vi "Main.vi"() -> ()   [LabVIEW 2015]
uses:
  TypDefs/Loop States.ctl
  TypDefs/Loop Data.ctl
panel:
  in  "device name":tag="myDAQ1"
  in  "Exit Button":bool
  in  "Start Button":bool
  out "Status":string
  in  "Clear Button":bool
  in  "Save Button":bool
  out "XY Graph":cluster{"X":dbl[], "Y":dbl[]}(graph)
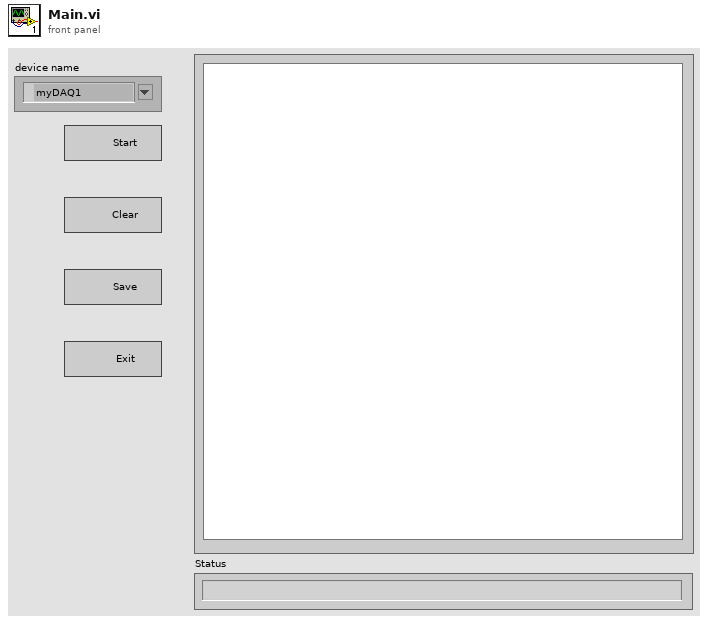
[diagram p1: front panel]
types:
  T1 = typedef "Loop Data.ctl" = cluster{"Status":string, "Graph Data":cluster{"X":dbl[], "Y":dbl[]}, "Recording Status":bool}
  T2 = typedef "Loop States.ctl" = enum16{"Error", "Wait for events", "Measure positions", "Update UI", "Initialization"}
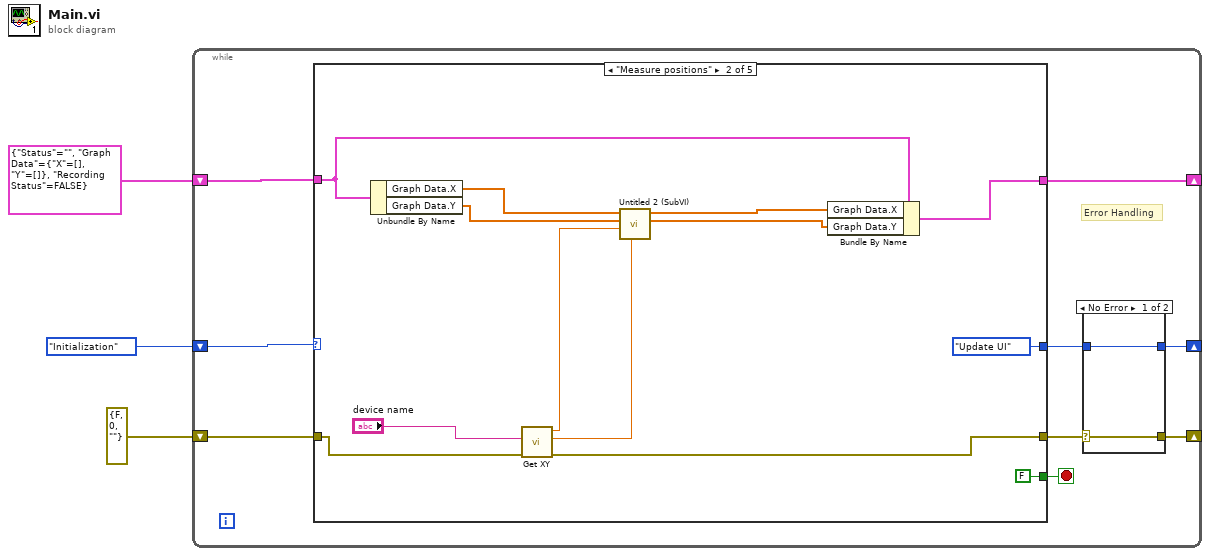
[diagram p0: block diagram]
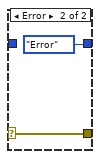
[diagram p2: hidden frame]
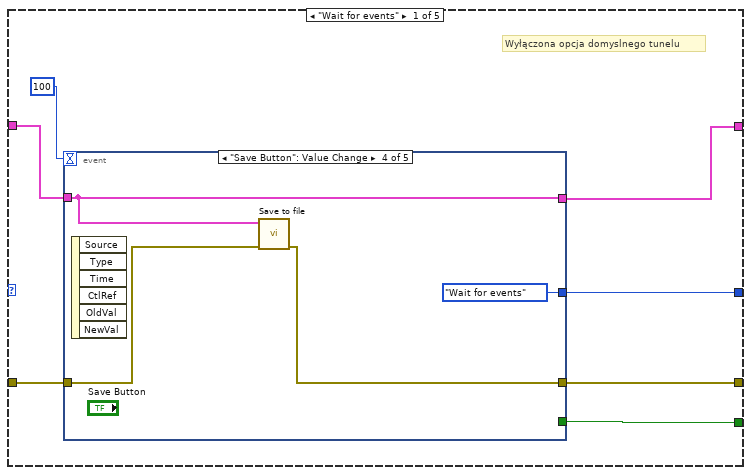
[diagram p3: hidden frame]
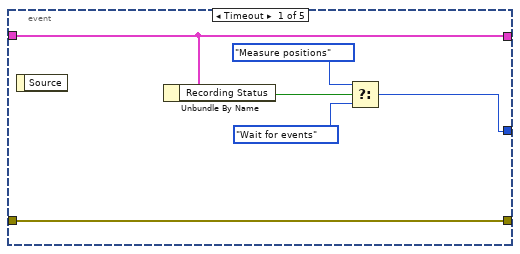
[diagram p4: hidden frame]
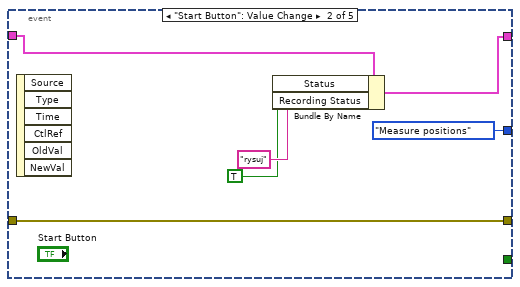
[diagram p5: hidden frame]
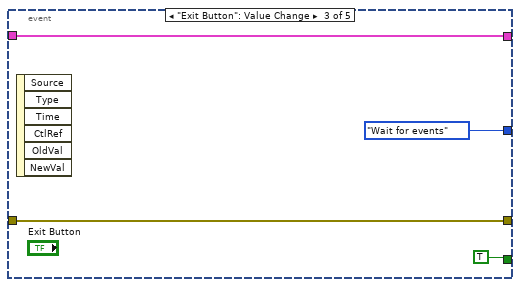
[diagram p6: hidden frame]
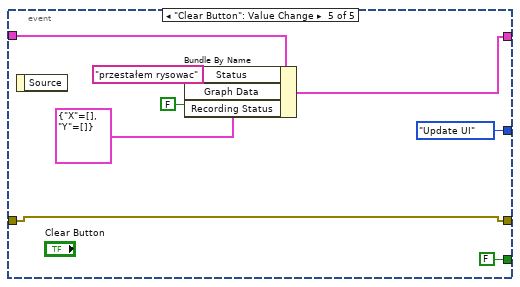
[diagram p7: hidden frame]
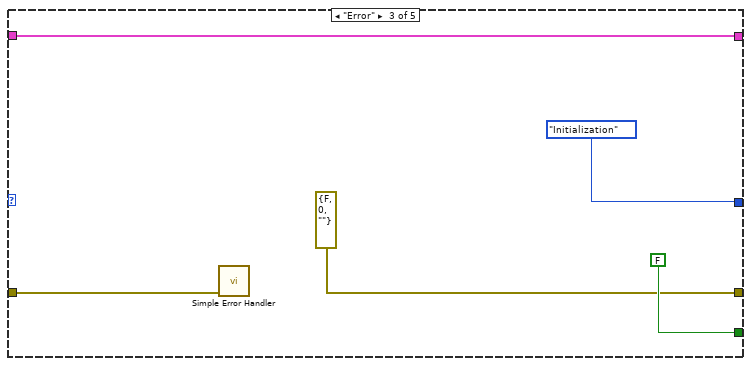
[diagram p8: hidden frame]
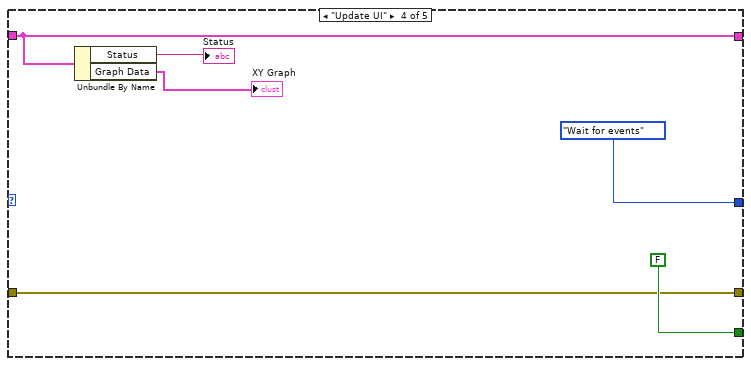
[diagram p9: hidden frame]
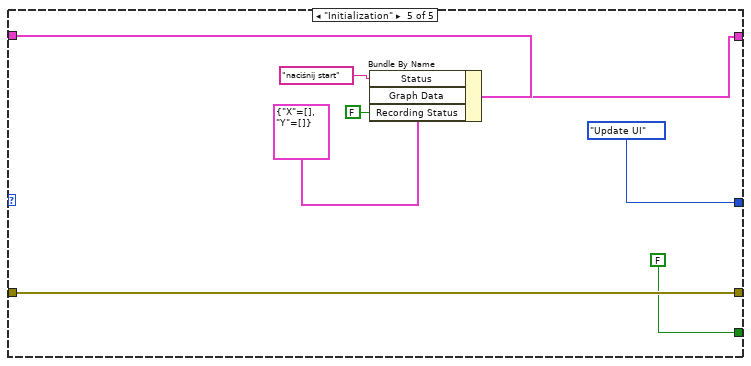
[diagram p10: hidden frame]
diagram:
  n1 = while {
    shift-right: [w10] -> _
    shift-left: T1 {"Status"="", "Graph Data"={"X"=[], "Y"=[]}, "Recording Status"=FALSE} -> [w11]
    shift-right: [w5] -> _
    shift-left: Loop_States."Initialization" -> [w12]
    shift-right: [w4] -> _
    shift-left: errorcluster {"status"=FALSE, "code"=0, "source"=""} ("error constant") -> [w8]
    stop <- w9 stop-if-true
    # "Error Handling"
    n2 = case shown="\"Measure positions\"" w12 {
      tunnel: w11 -> [w22 w61 w66 w71 w83]
      tunnel: [w20 w63 w66 w71 w82] -> w10
      tunnel: [w19 FALSE FALSE FALSE FALSE] -> w9
      tunnel: [w21 Loop_States."Update UI" Loop_States."Initialization" Loop_States."Wait for events" Loop_States."Update UI"] -> w6
      tunnel: w8 -> [w18 w60 w68 w74 w77]
      tunnel: [w17 w59 errorcluster {"status"=FALSE, "code"=0, "source"=""} ("error constant") w74 w77] -> w7
      frame "Wait for events" {
        # "Wyłączona opcja domyslnego tunelu"
        n3 = event shown="[3] \"Save Button\": Value Change" {
          selector: _ -> [_ _ _ _ _]
          dyn-events: _ -> [_ _ _ _ _]
          timeout: 100 -> [_ _ _ _ _]
          tunnel: w22 -> [w24 w35 w38 w42 w51]
          tunnel: [w25 Loop_States."Measure positions" Loop_States."Wait for events" Loop_States."Wait for events" Loop_States."Update UI"] -> w21
          tunnel: [w24 w31 w38 w42 w50] -> w20
          tunnel: [_ _ TRUE _ FALSE] -> w19
          tunnel: w18 -> [w29 w32 w36 w41 w45]
          tunnel: [w29 w32 w36 w40 w45] -> w17
          event Timeout {
            n4 = event-data() -> ()  [unwired: 1 in, 1 out]
            n5 = Unbundle By Name(w24) -> ("Recording Status"=w28:bool)
            n6 = Select(t=Loop_States."Measure positions", s=w28, f=Loop_States."Wait for events") -> (s? t:f=w25:T2)
          }
          event "Start Button": Value Change {
            n7 = event-data() -> ()  [unwired: 1 in, 6 out]
            n8 = Bundle By Name(cluster=w35, "Status"="rysuj", "Recording Status"=TRUE) -> (w31:T1)
          }
          event "Exit Button": Value Change {
            n9 = event-data() -> ()  [unwired: 1 in, 6 out]
          }
          event "Save Button": Value Change {
            n10 = event-data() -> ()  [unwired: 1 in, 6 out]
            n11 = call "Save to file.vi"("error in (no error)"=w41, "Loop Data"=w42) -> ("error out"=w40:errorcluster)  [unwired: 9 in]
          }
          event "Clear Button": Value Change {
            n12 = event-data() -> ()  [unwired: 1 in, 1 out]
            n13 = Bundle By Name(cluster=w51, "Status"="przestałem rysowac", "Graph Data"=cluster{"X":dbl[], "Y":dbl[]} {"X"=[], "Y"=[]}, "Recording Status"=FALSE) -> (w50:T1)
          }
        }
      }
      frame "Measure positions" {
        n14 = Unbundle By Name(w61) -> ("Graph Data.X"=w58:dbl[], "Graph Data.Y"=w56:dbl[])
        n15 = call "Get XY.vi"("error in"=w60, "device name"="device name") -> ("error out"=w59:errorcluster, "Y"=w55:dbl, "X"=w57:dbl)  [unwired: 7 in]
        n16 = call "Untitled 2 (SubVI).vi"("Y"=w55, "X"=w57, "Y 2"=w56, "X 2"=w58) -> ("Array"=w52:dbl[], "Array 2"=w53:dbl[])  [unwired: 6 in]
        n17 = Bundle By Name(cluster=w61, "Graph Data.X"=w53, "Graph Data.Y"=w52) -> (w63:T1)
      }
      frame "Error" {
        n18 = call <vilib>:"Simple Error Handler.vi"("error in (no error)"=w68) -> ()  [unwired: 4 in, 5 out]
      }
      frame "Update UI" {
        n19 = Unbundle By Name(w71) -> ("Status"=→"Status":string, "Graph Data"=→"XY Graph":cluster{"X":dbl[], "Y":dbl[]})
      }
      frame "Initialization" {
        n20 = Bundle By Name(cluster=w83, "Status"="naciśnij start", "Graph Data"=cluster{"X":dbl[], "Y":dbl[]} {"X"=[], "Y"=[]}, "Recording Status"=FALSE) -> (w82:T1)
      }
    }
    n21 = case shown="No Error" w7 {
      selector: w7 -> [w13 w15]
      tunnel: w6 -> [w14 _]
      tunnel: [w14 Loop_States."Error"] -> w5
      tunnel: [w13 w15] -> w4
      frame No Error {
      }
      frame Error {
      }
    }
  }
